vi "Мульт_мпа.vi"(10 "МПА":dbl(knob) scale=0.0..70.0) -> (2 "регулятор":dbl)   [LabVIEW 2018]
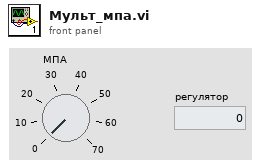
[diagram p1: front panel]
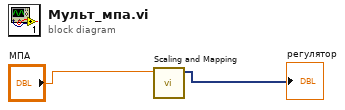
[diagram p0: block diagram]
diagram:
  n1 = call "Scaling and Mapping"("Signals"="МПА") -> ("Scaled Signals"=→"регулятор":dynamicdata)  [unwired: 9 in, 1 out]
